vi "Create Function String (Harmonics K).vi"(6 "Order (-1: Total)":i32=-1 min=-1 max=50 step=1, 8 "error in (no error)":errorcluster, 9 "Element (1: 1)":i32(ring)=1 items=["1"=1, "2"=2, "3"=3, "Sigma A"=4], 10 "Function (0: U(k))":i32(ring) items=["U(k)", "I(k)", "P(k)", "Lambda(k)", "Phi(k)", "PhiU(k)", "PhiI(k)", "Uhdf(k)", "Ihdf(k)", "Phdf(k)"], 11 "VISA resource name":refnum<visa-resource-name>) -> (0 "error out":errorcluster, 2 "Function String":string, 3 "VISA resource name out":refnum<visa-resource-name>)   [LabVIEW 2016, in "Yokogawa WT300 Series.lvlib"]
doc: "Create a harmonics(k) function string.\n\n<b>Note:</b>\nThis setting valid on models with the harmonic\nmeasurement (/G5) option."
uses:
  Yokogawa WT300 Series.lvlib
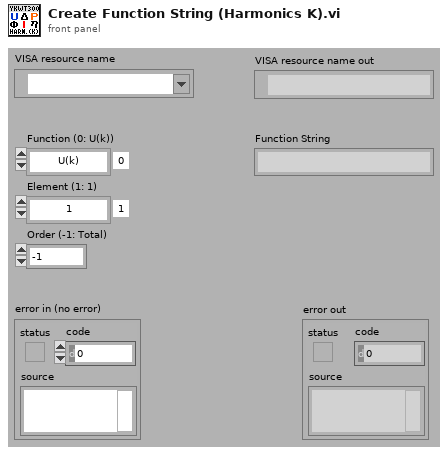
[diagram p1: front panel]
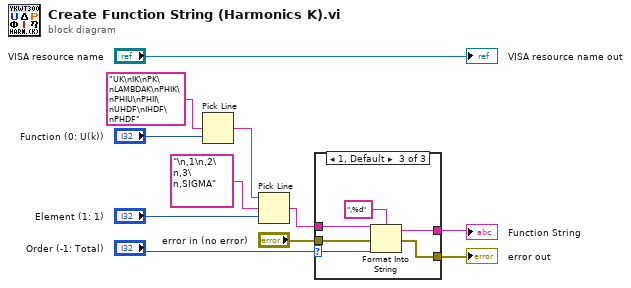
[diagram p0: block diagram]
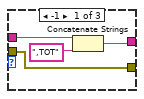
[diagram p2: hidden frame]
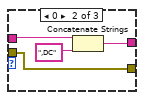
[diagram p3: hidden frame]
diagram:
  n1 = Pick Line ("ライン選択")(multi-line string="UK\nIK\nPK\nLAMBDAK\nPHIK\nPHIU\nPHII\nUHDF\nIHDF\nPHDF" ("複数行文字列"), line index="Function (0: U(k))") -> (output string=w7:string)  [unwired: 1 in]
  n2 = Pick Line ("ライン選択")(string ("")=w7, multi-line string="\n,1\n,2\n,3\n,SIGMA" ("複数行文字列"), line index="Element (1: 1)") -> (output string=w4:string)
  n3 = case shown="1, Default" "Order (-1: Total)" {
    selector: "Order (-1: Total)" -> [_ _ w23]
    tunnel: w4 -> [w14 w18 w24]
    tunnel: "error in (no error)" -> [w13 w17 w22]
    tunnel: [w13 w17 w21] -> w2
    tunnel: [w12 w16 w20] -> w1
    frame -1 {
      n4 = Concatenate Strings(w14, ",TOT" ("文字列")) -> (w12:string)
    }
    frame 0 {
      n5 = Concatenate Strings(w18, ",DC" ("文字列")) -> (w16:string)
    }
    frame 1, Default {
      n6 = Format Into String(format string=",%d" ("形式文字列"), initial string=w24, error in=w22, w23) -> (resulting string=w20:string, error out=w21:errorcluster)
    }
  }
  "error out" <- w2
  "Function String" <- w1
  "VISA resource name out" <- "VISA resource name"
